vi "Pins to NI-VNA Sessions.vi"(0 "Semiconductor Module Context":T1, 5 "Pins":string[](array[string]), 11 "error in (no error)":errorcluster) -> (2 "Pin Query Context":refnum<class "MultiplePinMultipleSessionQueryContext.lvclass">, 4 "Semiconductor Module Context Out":T1, 6 "Instrument Sessions":refnum<k15>[](array[refnum]), 10 "Channel Lists":string[](array[string]), 15 "error out":errorcluster)   [LabVIEW 2013, in "VNA Custom Instrument.lvlib"]
doc: "Returns NI-VNA sessions required to access one or more pins."
uses:
  VNA Custom Instrument.lvlib
  <vilib>/NI_TestStand_SemiconductorModule/NI_TestStand_Semiconductor_Module.lvlibp/PinMap/General/SemiconductorModuleContext.ctl
  <vilib>/NI_TestStand_SemiconductorModule/NI_TestStand_Semiconductor_Module.lvlibp/PinMap/PinQueryContext/MultiplePinMultipleSessionQueryContext/MultiplePinMultipleSessionQueryContext.lvclass
  <vilib>/NI_TestStand_SemiconductorModule/NI_TestStand_Semiconductor_Module.lvlibp
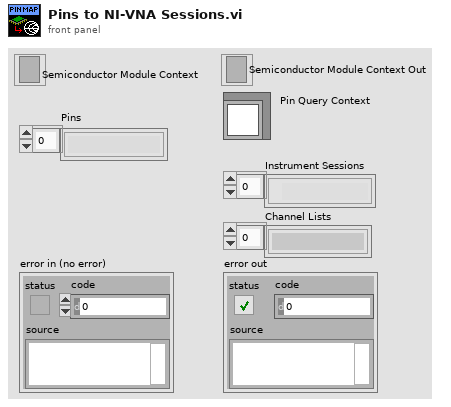
[diagram p1: front panel]
types:
  T1 = typedef "NI_TestStand_Semiconductor_Module.lvlibp/SemiconductorModuleContext.ctl" = refnum<k7>
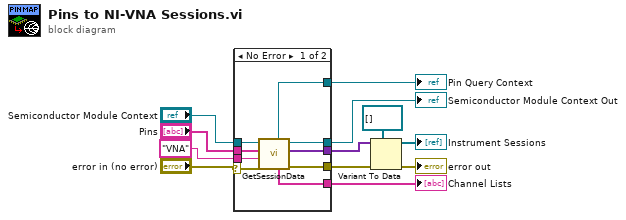
[diagram p0: block diagram]
diagram:
  n1 = case shown="No Error" "error in (no error)" {
    selector: "error in (no error)" -> [w13 w23]
    tunnel: "Semiconductor Module Context" -> [w21 w22]
    tunnel: "Pins" -> [w20 _]
    tunnel: "VNA" ("Instrument Type Id") -> [w19 _]
    tunnel: [w18 _] -> w9
    tunnel: [w17 w23] -> w8
    tunnel: [w16 _] -> w7
    tunnel: [w15 w22] -> w6
    tunnel: [w14 _] -> w2
    frame No Error {
      n2 = call <vilib>:"GetSessionData.vi"("error in (no error)"=w13, "Instrument Type Id"=w19, "Pins"=w20, "Semiconductor Module Context"=w21) -> ("error out"=w17:errorcluster, "Session Data"=w16:variant[], "Semiconductor Module Context Out"=w15:T1, "Channel Lists"=w18:string[], "Pin Query Context"=w14:refnum<class "MultiplePinMultipleSessionQueryContext.lvclass">)  [unwired: 2 in, 1 out]
    }
    frame Error {
    }
  }
  "Channel Lists" <- w9
  "Semiconductor Module Context Out" <- w6
  "Pin Query Context" <- w2
  n3 = Variant To Data(error in=w8, type=refnum<k15>[] [], Variant=w7) -> (data=→"Instrument Sessions":refnum<k15>[], error out=→"error out":errorcluster)
